vi "FdxReadBSPVersionCvi.vi"(8 "error in":errorcluster, 11 "InstrumentHandle_board in":u32) -> (0 "error out":errorcluster, 1 "BSP Version Out":T1, 3 "InstrumentHandle_board out":u32)   [LabVIEW 2020, in "AIM664LV.lvlib"]
doc: "This function returns the version numbers of all board software package components for the AIM board."
uses:
  AIM664LV.lvlib
  AFDX_LibraryAdmin/FdxGlobalDllPath.vi
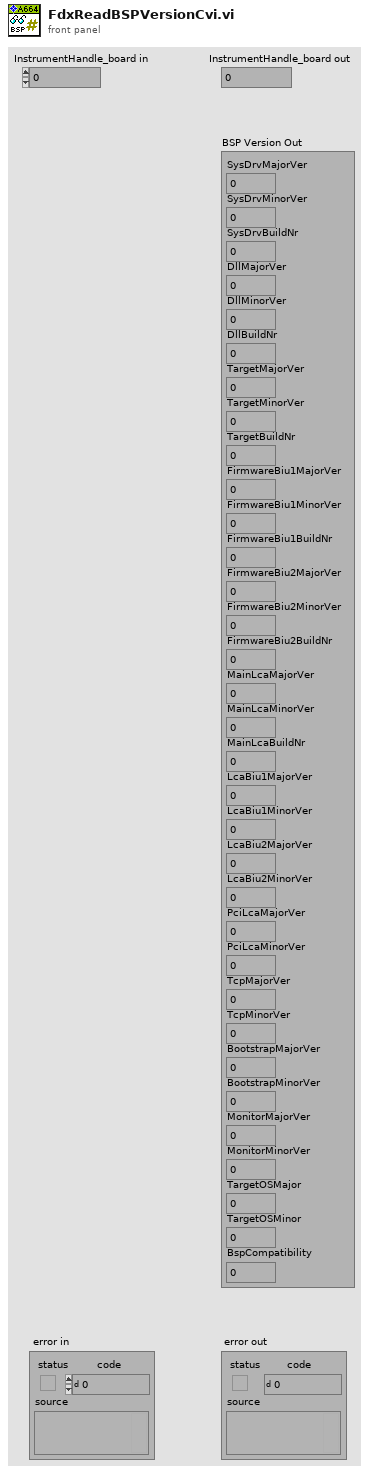
[diagram p1: front panel]
types:
  T1 = cluster{"SysDrvMajorVer":u32, "SysDrvMinorVer":u32, "SysDrvBuildNr":u32, "DllMajorVer":u32, "DllMinorVer":u32, "DllBuildNr":u32, "TargetMajorVer":u32, "TargetMinorVer":u32, "TargetBuildNr":u32, "FirmwareBiu1MajorVer":u32, "FirmwareBiu1MinorVer":u32, "FirmwareBiu1BuildNr":u32, "FirmwareBiu2MajorVer":u32, "FirmwareBiu2MinorVer":u32, "FirmwareBiu2BuildNr":u32, "MainLcaMajorVer":u32, "MainLcaMinorVer":u32, "MainLcaBuildNr":u32, "LcaBiu1MajorVer":u32, "LcaBiu1MinorVer":u32, "LcaBiu2MajorVer":u32, "LcaBiu2MinorVer":u32, "PciLcaMajorVer":u32, "PciLcaMinorVer":u32, "TcpMajorVer":u32, "TcpMinorVer":u32, "BootstrapMajorVer":u32, "BootstrapMinorVer":u32, "MonitorMajorVer":u32, "MonitorMinorVer":u32, "TargetOSMajor":u32, "TargetOSMinor":u32, "BspCompatibility":u32}
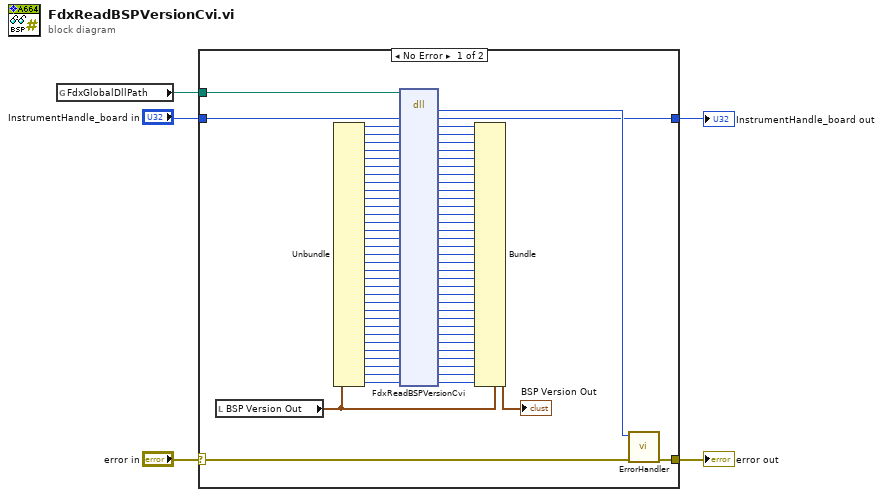
[diagram p0: block diagram]
diagram:
  n1 = global read "FdxGlobalDllPath.vi" "FdxGlobalDllPath"() -> (w3:path)
  n2 = case shown="No Error" "error in" {
    selector: "error in" -> [w78 w81]
    tunnel: [w79 w81] -> w5
    tunnel: w3 -> [w8 _]
    tunnel: "InstrumentHandle_board in" -> [w7 w80]
    tunnel: [w6 w80] -> w1
    frame No Error {
      n3 = local read "BSP Version Out"() -> (w9:T1)
      n4 = Unbundle(w9) -> ("SysDrvMajorVer"=w58:u32, "SysDrvMinorVer"=w57:u32, "SysDrvBuildNr"=w56:u32, "DllMajorVer"=w55:u32, "DllMinorVer"=w54:u32, "DllBuildNr"=w53:u32, "TargetMajorVer"=w52:u32, "TargetMinorVer"=w51:u32, "TargetBuildNr"=w50:u32, "FirmwareBiu1MajorVer"=w49:u32, "FirmwareBiu1MinorVer"=w48:u32, "FirmwareBiu1BuildNr"=w47:u32, "FirmwareBiu2MajorVer"=w46:u32, "FirmwareBiu2MinorVer"=w45:u32, "FirmwareBiu2BuildNr"=w44:u32, "MainLcaMajorVer"=w43:u32, "MainLcaMinorVer"=w42:u32, "MainLcaBuildNr"=w41:u32, "LcaBiu1MajorVer"=w40:u32, "LcaBiu1MinorVer"=w39:u32, "LcaBiu2MajorVer"=w38:u32, "LcaBiu2MinorVer"=w37:u32, "PciLcaMajorVer"=w36:u32, "PciLcaMinorVer"=w35:u32, "TcpMajorVer"=w34:u32, "TcpMinorVer"=w33:u32, "BootstrapMajorVer"=w32:u32, "BootstrapMinorVer"=w31:u32, "MonitorMajorVer"=w30:u32, "MonitorMinorVer"=w29:u32, "TargetOSMajor"=w28:u32, "TargetOSMinor"=w27:u32, "BspCompatibility"=w26:u32)
      n5 = dll-call lib="aim_fdx.19.dll" fn="FdxReadBSPVersionCvi"(path in=w8, "InstrumentHandle"=w7, "SysDrvMajorVer"=w58, "SysDrvMinorVer"=w57, "SysDrvBuildNr"=w56, "DllMajorVer"=w55, "DllMinorVer"=w54, "DllBuildNr"=w53, "TargetMajorVer"=w52, "TargetMinorVer"=w51, "TargetBuildNr"=w50, "FirmwareBiu1MajorVer"=w49, "FirmwareBiu1MinorVer"=w48, "FirmwareBiu1BuildNr"=w47, "FirmwareBiu2MajorVer"=w46, "FirmwareBiu2MinorVer"=w45, "FirmwareBiu2BuildNr"=w44, "MainLcaMajorVer"=w43, "MainLcaMinorVer"=w42, "MainLcaBuildNr"=w41, "LcaBiu1MajorVer"=w40, "LcaBiu1MinorVer"=w39, "LcaBiu2MajorVer"=w38, "LcaBiu2MinorVer"=w37, "PciLcaMajorVer"=w36, "PciLcaMinorVer"=w35, "TcpMajorVer"=w34, "TcpMinorVer"=w33, "BootstrapMajorVer"=w32, "BootstrapMinorVer"=w31, "MonitorMajorVer"=w30, "MonitorMinorVer"=w29, "TargetOSMajor"=w28, "TargetOSMinor"=w27, "BspCompatibility"=w26) -> ("status"=w77:i32, "InstrumentHandle"=w6:u32, "SysDrvMajorVer"=w76:u32, "SysDrvMinorVer"=w75:u32, "SysDrvBuildNr"=w74:u32, "DllMajorVer"=w73:u32, "DllMinorVer"=w72:u32, "DllBuildNr"=w71:u32, "TargetMajorVer"=w70:u32, "TargetMinorVer"=w69:u32, "TargetBuildNr"=w68:u32, "FirmwareBiu1MajorVer"=w67:u32, "FirmwareBiu1MinorVer"=w66:u32, "FirmwareBiu1BuildNr"=w65:u32, "FirmwareBiu2MajorVer"=w64:u32, "FirmwareBiu2MinorVer"=w63:u32, "FirmwareBiu2BuildNr"=w62:u32, "MainLcaMajorVer"=w61:u32, "MainLcaMinorVer"=w60:u32, "MainLcaBuildNr"=w25:u32, "LcaBiu1MajorVer"=w24:u32, "LcaBiu1MinorVer"=w23:u32, "LcaBiu2MajorVer"=w22:u32, "LcaBiu2MinorVer"=w21:u32, "PciLcaMajorVer"=w20:u32, "PciLcaMinorVer"=w19:u32, "TcpMajorVer"=w10:u32, "TcpMinorVer"=w18:u32, "BootstrapMajorVer"=w17:u32, "BootstrapMinorVer"=w16:u32, "MonitorMajorVer"=w15:u32, "MonitorMinorVer"=w14:u32, "TargetOSMajor"=w13:u32, "TargetOSMinor"=w12:u32, "BspCompatibility"=w11:u32)  [unwired: 2 in, 2 out]
      n6 = Bundle(cluster=w9, "SysDrvMajorVer"=w76, "SysDrvMinorVer"=w75, "SysDrvBuildNr"=w74, "DllMajorVer"=w73, "DllMinorVer"=w72, "DllBuildNr"=w71, "TargetMajorVer"=w70, "TargetMinorVer"=w69, "TargetBuildNr"=w68, "FirmwareBiu1MajorVer"=w67, "FirmwareBiu1MinorVer"=w66, "FirmwareBiu1BuildNr"=w65, "FirmwareBiu2MajorVer"=w64, "FirmwareBiu2MinorVer"=w63, "FirmwareBiu2BuildNr"=w62, "MainLcaMajorVer"=w61, "MainLcaMinorVer"=w60, "MainLcaBuildNr"=w25, "LcaBiu1MajorVer"=w24, "LcaBiu1MinorVer"=w23, "LcaBiu2MajorVer"=w22, "LcaBiu2MinorVer"=w21, "PciLcaMajorVer"=w20, "PciLcaMinorVer"=w19, "TcpMajorVer"=w10, "TcpMinorVer"=w18, "BootstrapMajorVer"=w17, "BootstrapMinorVer"=w16, "MonitorMajorVer"=w15, "MonitorMinorVer"=w14, "TargetOSMajor"=w13, "TargetOSMinor"=w12, "BspCompatibility"=w11) -> (→"BSP Version Out":T1)
      n7 = call "ErrorHandler.vi"("error in"=w78, "AIM Error"=w77) -> ("error out"=w79:errorcluster)  [unwired: 9 in]
    }
    frame Error {
    }
  }
  "error out" <- w5
  "InstrumentHandle_board out" <- w1
